vi "SavePathJson.vi"(10 "File Name":string=".csv", 11 "Path In":string="C:\\CS-BarCode\\Save Date\\") -> (3 "Folder Path":path, 5 "File Path":path)   [LabVIEW 2014]
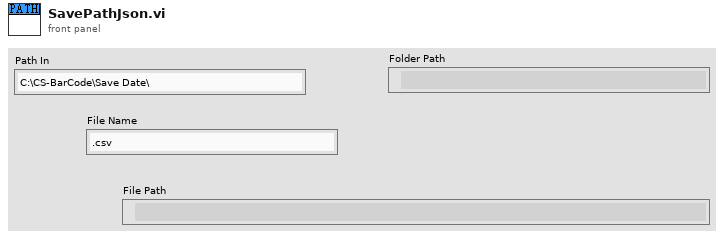
[diagram p1: front panel]
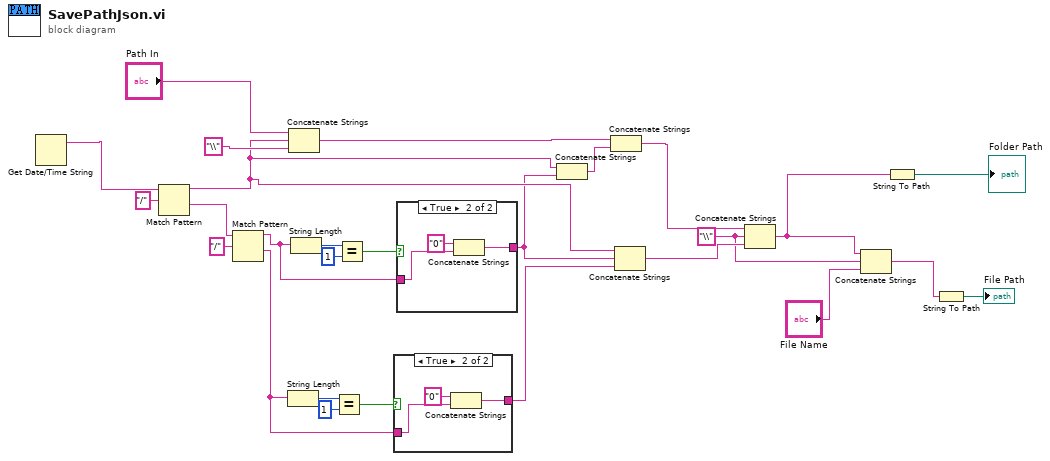
[diagram p0: block diagram]
diagram:
  w2 = "\\" ("string")
  n1 = Get Date/Time String() -> (date string=w27:string)  [unwired: 3 in, 1 out]
  n2 = Match Pattern(string=w27, regular expression="/") -> (before substring=w11:string, after substring=w23:string)  [unwired: 1 in, 2 out]
  n3 = Match Pattern(string=w23, regular expression="/") -> (before substring=w18:string, after substring=w12:string)  [unwired: 1 in, 2 out]
  n4 = String Length(string=w12) -> (length=w13:i32)
  n5 = Concatenate Strings("Path In", w11, "\\") -> (w17:string)
  n6 = String Length(string=w18) -> (length=w21:i32)
  n7 = Equal?(x=w13, y=1) -> (x = y?=w15:bool)
  n8 = Equal?(x=w21, y=1) -> (x = y?=w19:bool)
  n9 = case shown="True" w15 {
    tunnel: w12 -> [w28 w31]
    tunnel: [w28 w29] -> w9
    frame False {
    }
    frame True {
      n10 = Concatenate Strings("0" ("string"), w31) -> (w29:string)
    }
  }
  n11 = case shown="True" w19 {
    tunnel: w18 -> [w32 w35]
    tunnel: [w32 w33] -> w10
    frame False {
    }
    frame True {
      n12 = Concatenate Strings("0" ("string"), w35) -> (w33:string)
    }
  }
  n13 = Concatenate Strings(w11, w10) -> (w16:string)
  n14 = Concatenate Strings(w17, w16) -> (w7:string)
  n15 = Concatenate Strings(w11, w10, w9) -> (w8:string)
  n16 = Concatenate Strings(w7, w2, w8) -> (w1:string)
  n17 = Concatenate Strings(w1, w2, "File Name") -> (w3:string)
  n18 = String To Path(string=w1) -> (path=→"Folder Path":path)
  n19 = String To Path(string=w3) -> (path=→"File Path":path)
